vi "pp_shuffleRows.vi"(11 "Input":dbl[][](array[numeric])) -> (3 "Output":dbl[][](array[numeric]))   [LabVIEW 2013]
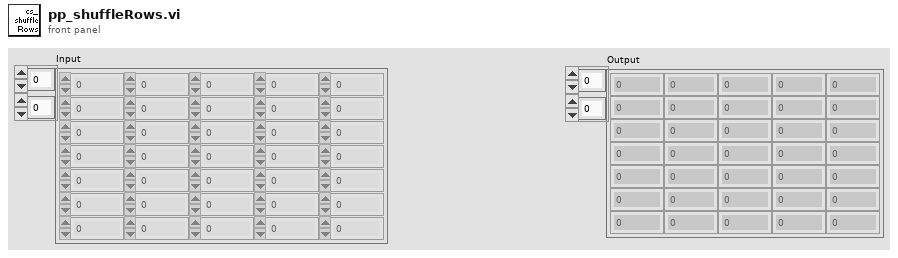
[diagram p1: front panel]
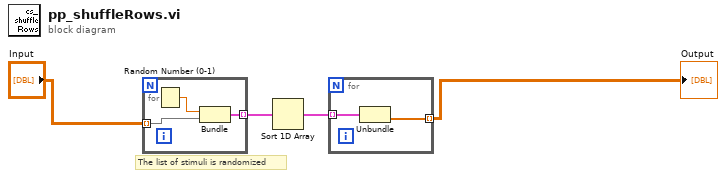
[diagram p0: block diagram]
diagram:
  # "The list of stimuli is randomized"
  n1 = for {
    tunnel: "Input" -> [w6] mode=indexing
    tunnel: [w5] -> w3 mode=indexing
    n2 = Random Number (0-1)() -> (number: 0 to 1=w7:dbl)
    n3 = Bundle("number: 0 to 1"=w7, "Input"=w6) -> (w5:cluster{"number: 0 to 1":dbl, "Input":dbl[]})  [unwired: 1 in]
  }
  n4 = Sort 1D Array(array=w3) -> (sorted array=w4:cluster{"number: 0 to 1":dbl, "Input":dbl[]}[])
  n5 = for {
    tunnel: w4 -> [w8] mode=indexing
    tunnel: [w9] -> w1 mode=indexing
    n6 = Unbundle(w8) -> ("Input"=w9:dbl[])  [unwired: 1 out]
  }
  "Output" <- w1
